vi "AutoInit.vi"   [LabVIEW 2020]
doc: "Set all robot instructions to their proper intial state."
uses:
  drivercommands.vi
  autonomousinfo.vi
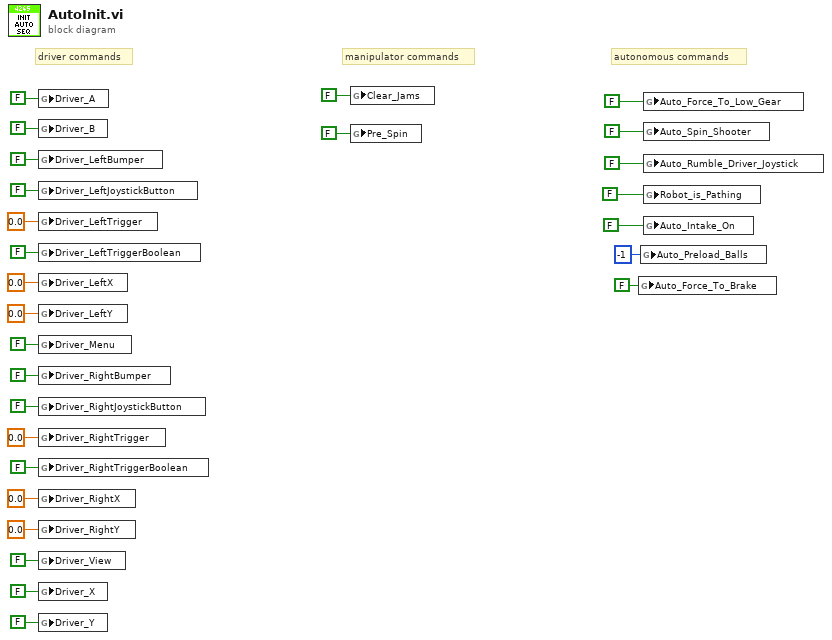
[diagram p0: block diagram]
diagram:
  # "manipulator commands"
  # "driver commands"
  # "autonomous commands"
  n1 = global write "drivercommands.vi" "Driver_A"(FALSE ("Driver_A")) -> ()
  n2 = global write "drivercommands.vi" "Driver_B"(FALSE ("Driver_B")) -> ()
  n3 = global write "drivercommands.vi" "Driver_LeftBumper"(FALSE ("Driver_LeftBumper")) -> ()
  n4 = global write "drivercommands.vi" "Driver_LeftJoystickButton"(FALSE ("Driver_LeftJoystickButton")) -> ()
  n5 = global write "drivercommands.vi" "Driver_LeftTrigger"(0.0 ("Driver_LeftTrigger")) -> ()
  n6 = global write "drivercommands.vi" "Driver_LeftTriggerBoolean"(FALSE ("Driver_LeftTriggerBoolean")) -> ()
  n7 = global write "drivercommands.vi" "Driver_LeftX"(0.0 ("Driver_LeftX")) -> ()
  n8 = global write "drivercommands.vi" "Driver_LeftY"(0.0 ("Driver_LeftY")) -> ()
  n9 = global write "drivercommands.vi" "Driver_Menu"(FALSE ("Driver_Menu")) -> ()
  n10 = global write "drivercommands.vi" "Driver_RightBumper"(FALSE ("Driver_RightBumper")) -> ()
  n11 = global write "drivercommands.vi" "Driver_RightJoystickButton"(FALSE ("Driver_RightJoystickButton")) -> ()
  n12 = global write "drivercommands.vi" "Driver_RightTrigger"(0.0 ("Driver_RightTrigger")) -> ()
  n13 = global write "drivercommands.vi" "Driver_RightTriggerBoolean"(FALSE ("Driver_RightTriggerBoolean")) -> ()
  n14 = global write "drivercommands.vi" "Driver_RightX"(0.0 ("Driver_RightX")) -> ()
  n15 = global write "drivercommands.vi" "Driver_RightY"(0.0 ("Driver_RightY")) -> ()
  n16 = global write "drivercommands.vi" "Driver_View"(FALSE ("Driver_View")) -> ()
  n17 = global write "drivercommands.vi" "Driver_X"(FALSE ("Driver_X")) -> ()
  n18 = global write "drivercommands.vi" "Driver_Y"(FALSE ("Driver_Y")) -> ()
  n19 = global write "drivercommands.vi" "Clear_Jams"(FALSE ("Clear_Jams")) -> ()
  n20 = global write "drivercommands.vi" "Pre_Spin"(FALSE ("Clear_Jams")) -> ()
  n21 = global write "autonomousinfo.vi" "Auto_Force_To_Brake"(FALSE ("Auto_Force_To_Brake")) -> ()
  n22 = global write "autonomousinfo.vi" "Auto_Preload_Balls"(-1 ("Auto_Preload_Balls")) -> ()
  n23 = global write "autonomousinfo.vi" "Auto_Force_To_Low_Gear"(FALSE ("Auto_Force_To_Low_Gear")) -> ()
  n24 = global write "autonomousinfo.vi" "Auto_Spin_Shooter"(FALSE ("Auto_Force_To_Low_Gear")) -> ()
  n25 = global write "autonomousinfo.vi" "Auto_Rumble_Driver_Joystick"(FALSE ("Auto_Force_To_Low_Gear")) -> ()
  n26 = global write "autonomousinfo.vi" "Robot_is_Pathing"(FALSE ("Robot_is_Pathing")) -> ()
  n27 = global write "autonomousinfo.vi" "Auto_Intake_On"(FALSE ("Robot_is_Pathing")) -> ()
